vi "source to integer value.vi"(8 "error in (no error)":errorcluster caption="에러 입력(에러 없음)", 11 "WAV File 입력":refnum<class "WAV File.lvclass">) -> (0 "error out":errorcluster caption="에러 출력", 2 "integer value":dbl[](array[numeric]), 3 "WAV File 출력":refnum<class "WAV File.lvclass">)   [LabVIEW 2020, in "WAV File.lvclass"]
uses:
  WAV File.lvclass
  WAV File.lvclass/WAV File.ctl
  Waveform File/Waveform File.lvclass/Waveform File.ctl
  Accessors/Read sound format.vi
  Waveform File/Accessors/Read source waveform.vi
  Waveform File/Accessors/Read channel.vi
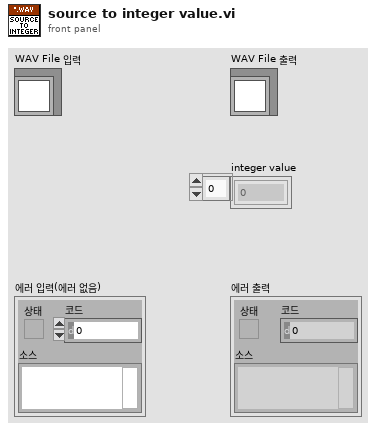
[diagram p1: front panel]
types:
  T1 = typedef "Sound Data Format.ctl" = cluster{"sample rate (S/s)":dbl, "number of channels":i32, "bits per sample":i32}
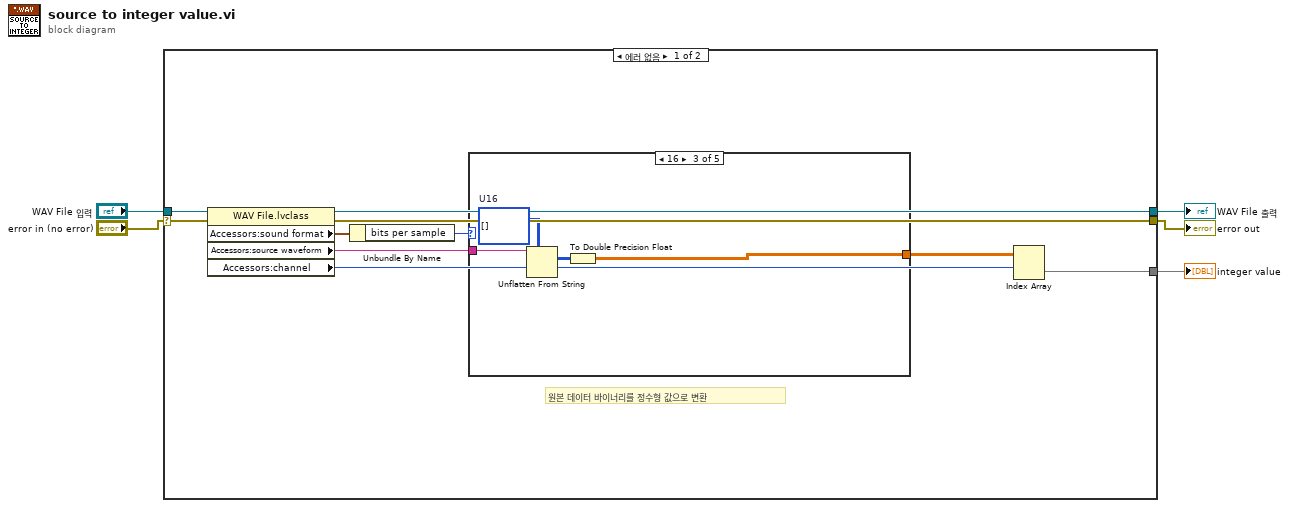
[diagram p0: block diagram]
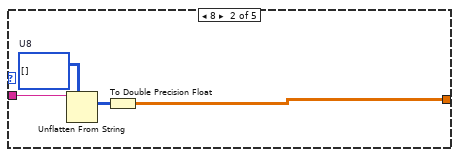
[diagram p3: hidden frame]
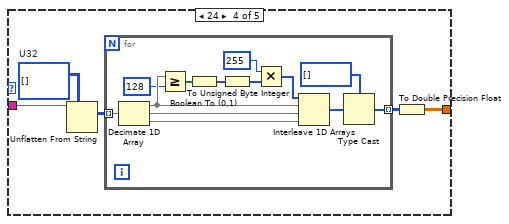
[diagram p4: hidden frame]
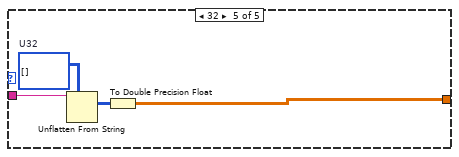
[diagram p5: hidden frame]
diagram:
  n1 = case shown="에러 없음" "error in (no error)" {
    selector: "error in (no error)" -> [w12 w47]
    tunnel: [w10 w47] -> w2
    tunnel: "WAV File 입력" -> [w15 w46]
    tunnel: [w14 w46] -> w4
    tunnel: [w8 _] -> w1
    frame No Error {
      # "원본 데이터 바이너리를 정수형 값으로 변환"
      n2 = property class="WAV File.lvclass"(reference=w15, error in=w12) -> (reference out=w14:refnum<class "WAV File.lvclass">, error out=w10:errorcluster, "Accessors:sound format"=w13:T1, "Accessors:source waveform"=w11:string, "Accessors:channel"=w7:i32)
      n3 = Unbundle By Name(w13) -> ("bits per sample"=w6:i32)
      n4 = case shown="16" w6 {
        tunnel: w11 -> [_ w19 w23 w28 w45]
        tunnel: [_ w16 w20 w24 w42] -> w9
        frame 0, Default {
        }
        frame 8 {
          w18 = u8[][] []  # U8
          n5 = Unflatten From String(type=w18, binary string=w19) -> (value=w17:u8[][])  [unwired: 3 in, 2 out]
          n6 = To Double Precision Float(number=w17) -> (double precision float=w16:dbl[][])
        }
        frame 16 {
          w22 = i16[][] []  # U16
          n7 = Unflatten From String(type=w22, binary string=w23) -> (value=w21:i16[][])  [unwired: 3 in, 2 out]
          n8 = To Double Precision Float(number=w21) -> (double precision float=w20:dbl[][])
        }
        frame 24 {
          w27 = u8[][] []  # U32
          n9 = Unflatten From String(type=w27, binary string=w28) -> (value=w26:u8[][])  [unwired: 3 in, 2 out]
          n10 = for {
            tunnel: w26 -> [w41] mode=indexing
            tunnel: [w29] -> w25 mode=indexing
            n11 = Decimate 1D Array(w41) -> (w38:u8[], w40:u8[], w39:u8[])
            n12 = Greater Or Equal?(x=w38, y=u8 128) -> (x >= y?=w36:bool[])
            n13 = Boolean To (0,1)(Boolean=w36) -> (0, 1=w35:i16[])
            n14 = To Unsigned Byte Integer(number=w35) -> (unsigned 8bit integer=w34:u8[])
            n15 = Multiply(x=u8 255, y=w34) -> (x*y=w32:u8[])
            n16 = Interleave 1D Arrays(w32, w38, w40, w39) -> (w31:u8[])
            n17 = Type Cast(type=i32[] [], x=w31) -> (*(type *) &x=w29:i32[])
          }
          n18 = To Double Precision Float(number=w25) -> (double precision float=w24:dbl[][])
        }
        frame 32 {
          w44 = i32[][] []  # U32
          n19 = Unflatten From String(type=w44, binary string=w45) -> (value=w43:i32[][])  [unwired: 3 in, 2 out]
          n20 = To Double Precision Float(number=w43) -> (double precision float=w42:dbl[][])
        }
      }
      n21 = Index Array(array=w9, index (row)=w7) -> (element=w8:dbl[])  [unwired: 1 in]
    }
    frame Error {
    }
  }
  "error out" <- w2
  "WAV File 출력" <- w4
  "integer value" <- w1
